vi "Dispose.vi"(8 "error in (no error)":errorcluster, 11 "ConcreteCreatorA in":refnum<class "ConcreteCreatorB.lvclass">) -> (0 "error out":errorcluster)   [LabVIEW 2020, in "FactoryMethod.lvlib" / "ConcreteCreatorB.lvclass"]
uses:
  ConcreteCreatorB.lvclass
  E:/GitHub/Design-Patterns-GoF_-_NI-LV/Creational/FactoryMethod/Base_Example/Creator/Creator.lvclass
  ConcreteProductB/ConcreteProductB.lvclass
  Creator/Creator.lvclass/Creator.ctl
  Creator/Private/Property/Product/Read Product.vi
  Product/Product.lvclass
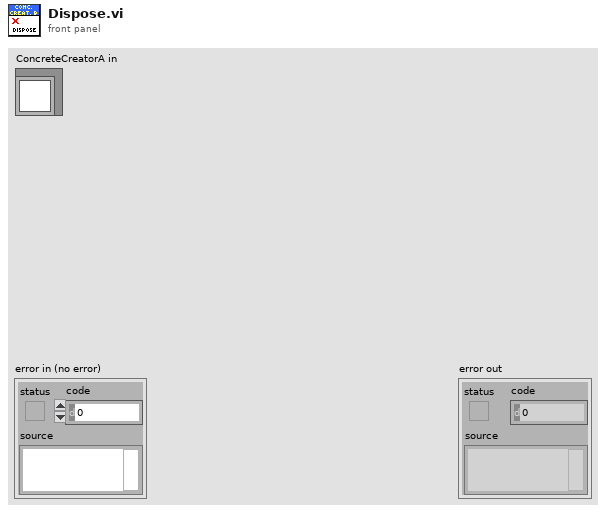
[diagram p1: front panel]
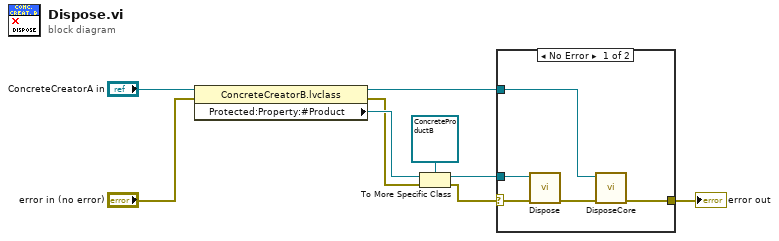
[diagram p0: block diagram]
diagram:
  n1 = property class="ConcreteCreatorB.lvclass"(reference="ConcreteCreatorA in", error in="error in (no error)") -> (reference out=w7:refnum<class "ConcreteCreatorB.lvclass">, error out=w2:errorcluster, "Protected:Property:#Product"=w5:refnum<class "Product.lvclass">)
  n2 = To More Specific Class(target class=refnum<class "ConcreteProductB.lvclass"> refnum ("ConcreteProductA in"), reference=w5, error in=w2) -> (specific class reference=w3:refnum<class "ConcreteProductB.lvclass">, error out=w1:errorcluster)
  n3 = case shown="No Error" w1 {
    selector: w1 -> [w11 w15]
    tunnel: [w14 w15] -> w9
    tunnel: w7 -> [w13 _]
    tunnel: w3 -> [w12 _]
    frame No Error {
      n4 = call "Dispose.vi"("error in (no error)"=w11, "ConcreteProductA in"=w12) -> ("error out"=w10:errorcluster)  [unwired: 9 in]
      n5 = call-dynamic "DisposeCore.vi"("error in (no error)"=w10, "ConcreteCreatorA in"=w13) -> ("error out"=w14:errorcluster)  [unwired: 8 in, 1 out]
    }
    frame Error {
    }
  }
  "error out" <- w9
